vi "To JSON.vi"(8 "error in":errorcluster, 11 "TPDO Communication Parameter in":refnum<class "TPDO Communication Parameter.lvclass">) -> (0 "error out":errorcluster, 2 "<JSON>":string, 3 "TPDO Communication Parameter out":refnum<class "TPDO Communication Parameter.lvclass">)   [LabVIEW 2020, in "CANopen.lvlib" / "TPDO Communication Parameter.lvclass"]
uses:
  TPDO Communication Parameter.lvclass
  TPDO Communication Parameter.lvclass/TPDO Communication Parameter.ctl
  b38e9efc-6aa8-4577-9f4e-d3ea1adb2934.vi
  <vilib>/JDP Science/JSONtext/JSONtext.lvlib
  PDO Communication Parameter/PDO Communication Parameter.lvclass
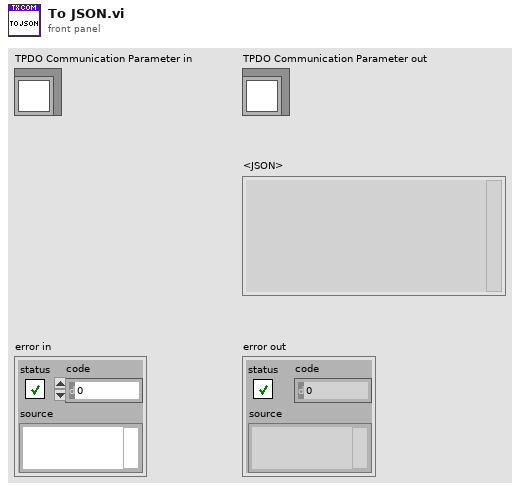
[diagram p1: front panel]
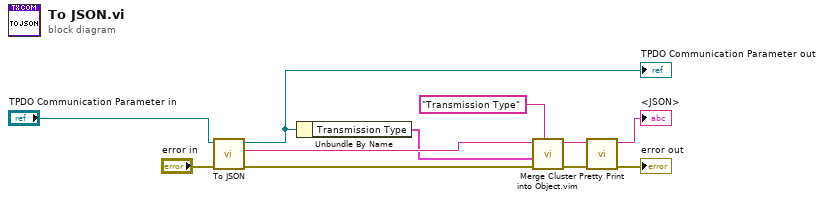
[diagram p0: block diagram]
diagram:
  n1 = call-parent "To JSON.vi"("error in"="error in", "PDO Communication Parameter in"="TPDO Communication Parameter in") -> ("error out"=w9:errorcluster, "<JSON>"=w7:string, "PDO Communication Parameter out"=w5:refnum<class "TPDO Communication Parameter.lvclass">)  [unwired: 7 in]
  "TPDO Communication Parameter out" <- w5
  n2 = Unbundle By Name(w5) -> ("Transmission Type"=w4:cluster{"Null":bool, "Value":u8})
  n3 = call "Merge Cluster into Object.vim"("$Path or Item Name"="Transmission Type", "error in (no error)"=w9, "Any Cluster"=w4, "JSON"=w7) -> ("error out"=w8:errorcluster, "<JSON>"=w2:string)  [unwired: 5 in]
  n4 = call <vilib>:"Pretty Print.vi"("error in (no error)"=w8, "JSON"=w2) -> ("error out"=→"error out":errorcluster, "<JSON>"=→"<JSON>":string)  [unwired: 7 in, 1 out]
